vi "boolean_trigger.vi"(11 "Input":bool) -> (3 "Rising Edge":bool)   [LabVIEW 2011]
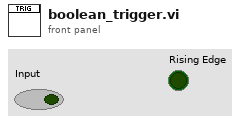
[diagram p1: front panel]
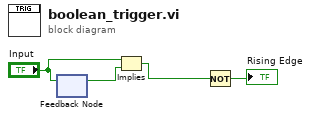
[diagram p0: block diagram]
diagram:
  n1 = feedback-in #1("Input") -> ()
  n2 = feedback #1() -> (w1:bool)  [unwired: 1 in]
  n3 = Implies(1:w1, 2:"Input") -> (0:w3:bool)
  n4 = Not(x=w3) -> (.not. x?=→"Rising Edge":bool)
